vi "FPGA Write.vi"(0 "FPGA VI Reference IN":refnum<k20>, 1 "Laser Signal Timing IN":i16[](array[numeric]), 2 "ephys_clock_timing IN":T1, 3 "frame_clock_timing IN":T1, 5 "Triggers IN":bool[](array[boolean]), 9 "Water Valve ON Time IN":i32, 11 "Error IN":errorcluster, 12 "Analog Outputs IN":sgl[](array[numeric])) -> (4 "FPGA VI Reference OUT":refnum<k20>, 15 "Error OUT":errorcluster)   [LabVIEW 2018]
uses:
  <vilib>/Utility/error.llb/Error Cluster From Error Code.vi
  <vilib>/rvi/errors/niLvFpgaAdjustHostInterfaceError.vi
  <vilib>/rvi/interface/nirviReadWriteControl/nirviReadWriteControl.xnode
  NiFpgaLv.dll
  <vilib>/rvi/interface/Simulation/niFpgaSimulationCallBeginRW.vi
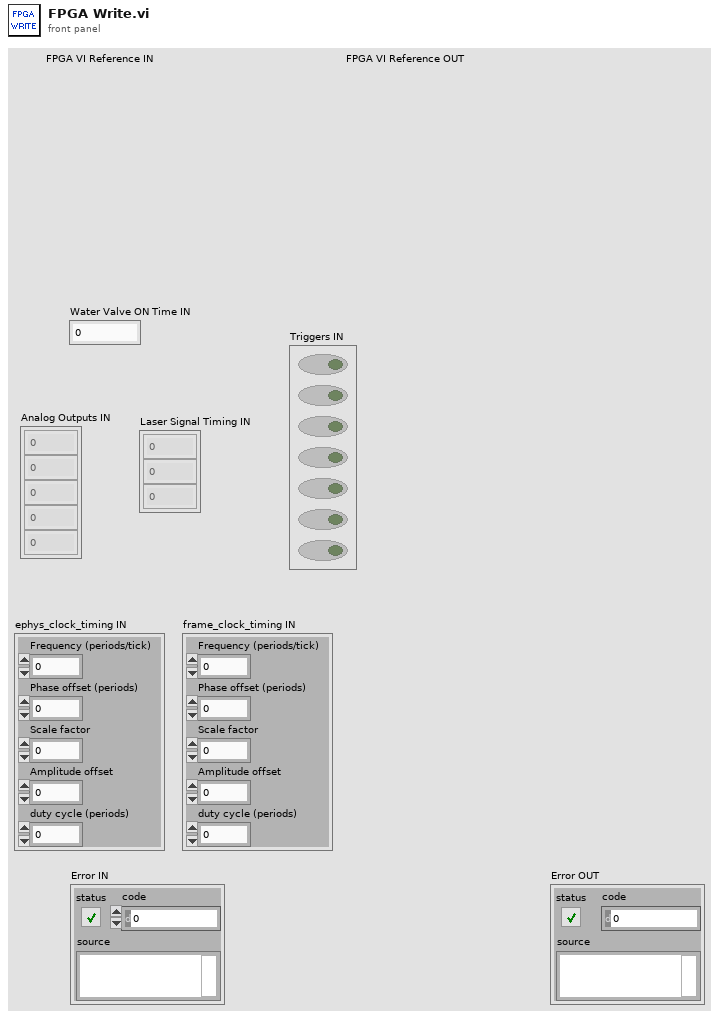
[diagram p1: front panel]
types:
  T1 = cluster{"Frequency (periods/tick)":fxp<+,32,0>, "Phase offset (periods)":fxp<+,32,0>, "Scale factor":fxp<+/-,16,1>, "Amplitude offset":fxp<+/-,16,16>, "duty cycle (periods)":fxp<+,32,0>}
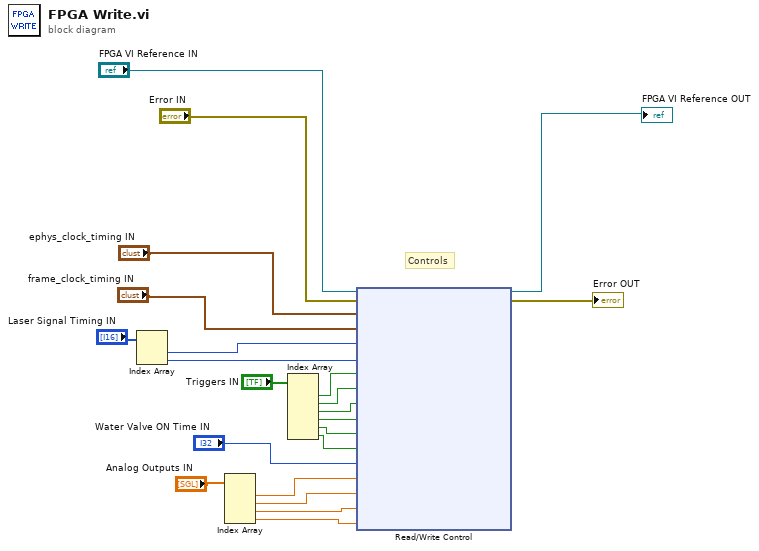
[diagram p0: block diagram]
diagram:
  # "Controls"
  n1 = Index Array(array="Laser Signal Timing IN") -> (element #1=w20:i16, element #2=w21:i16)  [unwired: 2 in]
  n2 = Index Array(array="Analog Outputs IN") -> (element #1=w6:sgl, element #2=w7:sgl, element #3=w8:sgl, element #4=w9:sgl)  [unwired: 4 in]
  n3 = Index Array(array="Triggers IN") -> (element #1=w14:bool, element #2=w15:bool, element #3=w16:bool, element #4=w17:bool, element #5=w18:bool, element #6=w22:bool)  [unwired: 6 in]
  n4 = xnode "Read/Write Control"("FPGA VI Reference In"="FPGA VI Reference IN", "error in"="Error IN", "ephys_clock_timing"="ephys_clock_timing IN", "frame_clock_timing"="frame_clock_timing IN", "laser_trig__ON Time"=w20, "laser_trig__OFF Time"=w21, "trial_ephys_ctrl"=w14, "whisker_video_ctrl"=w15, "right_texture_ctrl"=w16, "left_texture_ctrl"=w17, "water_valve_ctrl"=w18, "laser_ctrl"=w22, "water_valve_ctrl_ON Time"="Water Valve ON Time IN", "left_wall_AO"=w6, "right_wall_AO"=w7, "AO2"=w8, "laser_AO"=w9) -> ("FPGA VI Reference Out"=→"FPGA VI Reference OUT":refnum<k20>, "error out"=→"Error OUT":errorcluster)
